vi "Analysis.Build List of Unique Dates.vi"(10 "Date In":timestamp, 11 "Dates In":timestamp[](array[timestamp])) -> (2 "Added":bool, 3 "Dates Out":timestamp[](array[timestamp]), 5 "Index":i32)   [LabVIEW 2024]
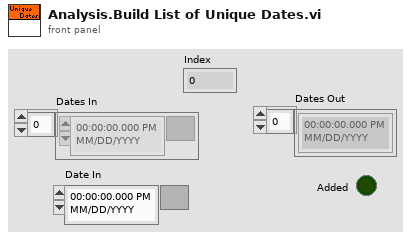
[diagram p1: front panel]
types:
  T1 = typedef "LVDateTimeRec.ctl" = cluster{"fractional second":dbl, "second":i32, "minute":i32, "hour":i32, "day of month":i32, "month":i32, "year":i32, "day of week":i32, "day of year":i32, "DST":i32}
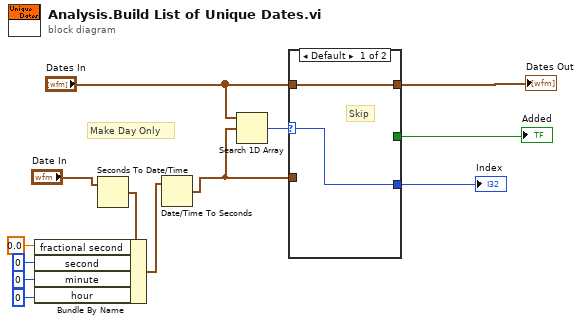
[diagram p0: block diagram]
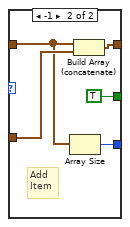
[diagram p2: hidden frame]
diagram:
  # "Make Day Only"
  n1 = Seconds To Date/Time(time stamp (now)="Date In") -> (date time rec=w7:T1)  [unwired: 1 in]
  n2 = Bundle By Name(cluster=w7, "fractional second"=0.0, "second"=0, "minute"=0, "hour"=0) -> (w2:T1)
  n3 = Date/Time To Seconds(2:w2) -> (0:w1:timestamp)  [unwired: 1 in]
  n4 = Search 1D Array(1D array="Dates In", element=w1) -> (index of element=w11:i32)  [unwired: 1 in]
  n5 = case shown="Default" w11 {
    selector: w11 -> [w14 _]
    tunnel: w1 -> [_ w19]
    tunnel: "Dates In" -> [w15 w16]
    tunnel: [w15 w20] -> w13
    tunnel: [_ TRUE] -> w10
    tunnel: [w14 w17] -> w9
    frame Default {
      # "Skip"
    }
    frame -1 {
      # "Add\nItem"
      n6 = Array Size(array=w16) -> (size(s)=w17:i32)
      n7 = Build Array (concatenate)(w16, w19) -> (w20:timestamp[])
    }
  }
  "Dates Out" <- w13
  "Added" <- w10
  "Index" <- w9
